vi "Set cif_plugincore_FifoStatistics.vi"(7 "Complete Call (T)":bool=TRUE, 8 "error in (no error)":errorcluster, 10 "package_templatemessage":T1, 11 "gRPCid":T3) -> (0 "error out":errorcluster)   [LabVIEW 2021, in "CIF_Launcher_server.lvlib"]
uses:
  CIF_Launcher_server.lvlib
  <vilib>/gRPC/LabVIEW gRPC Library/Shared/grpcId.ctl
  cif_plugincore_FifoStatistics.ctl
  cif_common_TimingStats.ctl
  cif_plugincore_FifoStatistics_Flat.ctl
  cif_common_TimingStats_Flat.ctl
  dcc74a39-081a-4bdd-860b-8ed792803c96.vi
  RichToFlatcif_common_TimingStats.vi
  <vilib>/gRPC/LabVIEW gRPC Library/Shared/TranslateGrpcError.vi
  <vilib>/gRPC/LabVIEW gRPC Library/Server API/Server/Get Server DLL Path.vi
  <vilib>/Utility/error.llb/Error Cluster From Error Code.vi
  <vilib>/gRPC/LabVIEW gRPC Library/grpc-lvsupport-release.lvlib
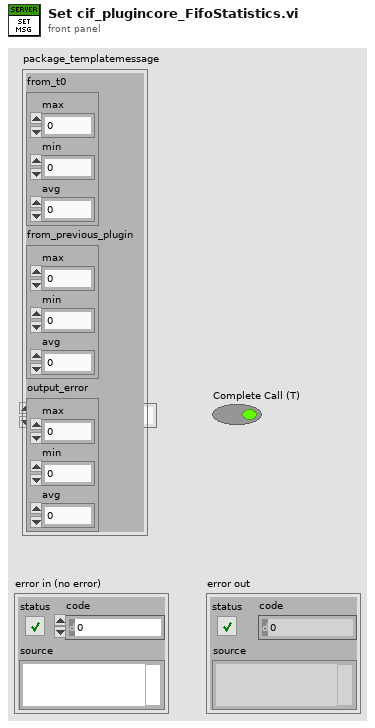
[diagram p1: front panel]
types:
  T1 = typedef "CIF_Launcher_server.lvlib/cif_plugincore_FifoStatistics.ctl" = cluster{"from_t0":T2, "from_previous_plugin":T2, "output_error":T2}
  T2 = typedef "CIF_Launcher_server.lvlib/cif_common_TimingStats.ctl" = cluster{"max":i64, "min":i64, "avg":dbl}
  T3 = typedef "grpc-lvsupport-release.lvlib/grpcId.ctl" = u64
  T4 = typedef "CIF_Launcher_server.lvlib/cif_plugincore_FifoStatistics_Flat.ctl" = cluster{"from_t0":T5, "from_previous_plugin":T5, "output_error":T5}
  T5 = typedef "CIF_Launcher_server.lvlib/cif_common_TimingStats_Flat.ctl" = cluster{"max":i64, "min":i64, "avg":dbl}
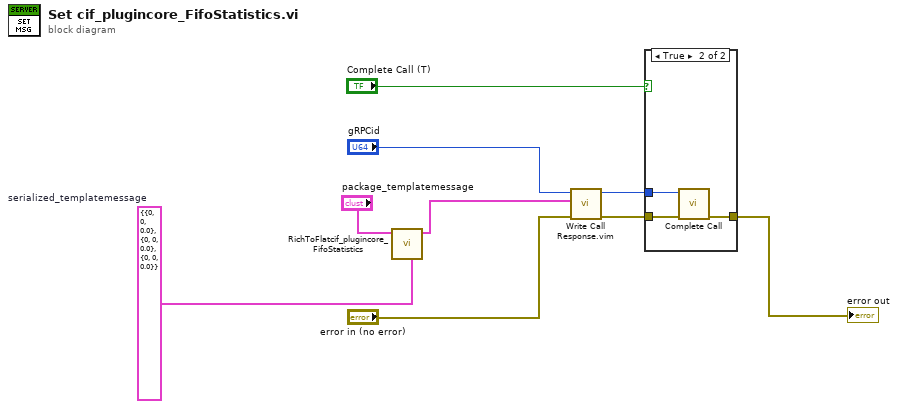
[diagram p0: block diagram]
diagram:
  w2 = T4 {"from_t0"={"max"=0, "min"=0, "avg"=0.0}, "from_previous_plugin"={"max"=0, "min"=0, "avg"=0.0}, "output_error"={"max"=0, "min"=0, "avg"=0.0}}  # serialized_templatemessage
  n1 = call "RichToFlatcif_plugincore_FifoStatistics.vi"("OutputClusterType"=w2, "InputCluster"="package_templatemessage") -> ("OutputCluster"=w1:T4)  [unwired: 9 in]
  n2 = call "Write Call Response.vim"("error in"="error in (no error)", "Response Data"=w1, "gRPCid in"="gRPCid") -> ("error out"=w6:errorcluster, "gRPCid out"=w7:T3)  [unwired: 7 in]
  n3 = case shown="True" "Complete Call (T)" {
    tunnel: [w10 w13] -> w9
    tunnel: w7 -> [_ w12]
    tunnel: w6 -> [w10 w11]
    frame False {
    }
    frame True {
      n4 = call <vilib>:"Complete Call.vi"("gRPCid"=w12, "error in"=w11) -> ("error out"=w13:errorcluster)  [unwired: 8 in]
    }
  }
  "error out" <- w9
